vi "checkBeginTestPlay.vi"(8 "error in (no error)":errorcluster, 10 "Game":refnum<class "Game.lvclass">, 11 "TestPlay in":refnum<class "TestPlay.lvclass">) -> (0 "error out":errorcluster, 1 "Test":bool, 2 "Score out":dbl, 3 "TestPlay out":refnum<class "TestPlay.lvclass">)   [LabVIEW 2021, in "TestPlay.lvclass"]
uses:
  TestPlay.lvclass
  Game_class/Game.lvclass
panel:
  in  "Score in":dbl=1.0 format="%#_13g"
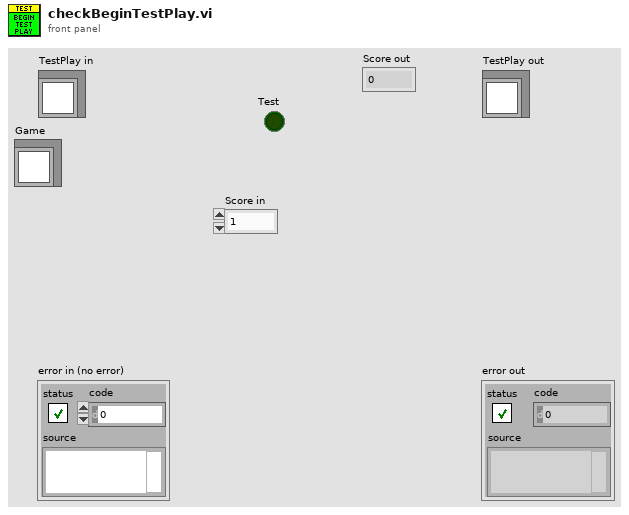
[diagram p1: front panel]
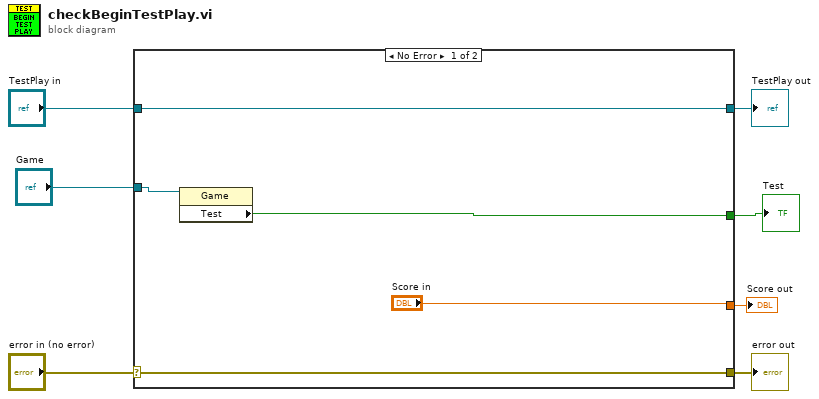
[diagram p0: block diagram]
diagram:
  n1 = case shown="No Error" "error in (no error)" {
    selector: "error in (no error)" -> [w11 w14]
    tunnel: [w11 w14] -> w6
    tunnel: [w12 w13] -> w4
    tunnel: "TestPlay in" -> [w12 w13]
    tunnel: "Game" -> [w10 _]
    tunnel: [w9 _] -> w2
    tunnel: ["Score in" _] -> w1
    frame No Error {
      n2 = property class="Game"(reference=w10) -> ("Test"=w9:bool)  [unwired: 1 in, 2 out]
    }
    frame Error {
    }
  }
  "error out" <- w6
  "TestPlay out" <- w4
  "Test" <- w2
  "Score out" <- w1
